vi "_Set Default.vi"   [LabVIEW 2012]
uses:
  <vilib>/eio/EIONode/EIONode.xnode
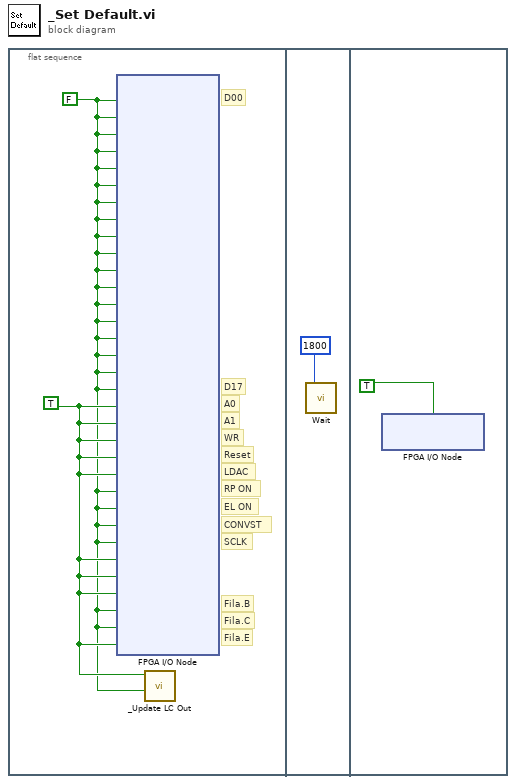
[diagram p0: block diagram]
diagram:
  n1 = flat-sequence {
    frame #0 {
      w2 = TRUE
      w1 = FALSE ("Port4/DIO8")
      # "Fila.E"
      # "Fila.C"
      # "Fila.B"
      # "SCLK"
      # "CONVST"
      # "EL ON"
      # "RP ON"
      # "LDAC"
      # "WR"
      # "A1"
      # "A0"
      # "Reset"
      # "D17"
      # "D00"
      n2 = xnode "FPGA I/O Node"("Port4/DIO8"=w1, "Port4/DIO7"=w1, "Port4/DIO6"=w1, "Port4/DIO5"=w1, "Port4/DIO4"=w1, "Port4/DIO3"=w1, "Port4/DIO2"=w1, "Port4/DIO1"=w1, "Port4/DIO0"=w1, "Port3/DIO8"=w1, "Port3/DIO7"=w1, "Port3/DIO6"=w1, "Port3/DIO5"=w1, "Port3/DIO4"=w1, "Port3/DIO3"=w1, "Port3/DIO2"=w1, "Port3/DIO1"=w1, "Port3/DIO0"=w1, "Port7/DIO1"=w2, "Port7/DIO0"=w2, "Port7/DIO3"=w2, "Port1/DIO4"=w2, "Port7/DIO2"=w2, "Port1/DIO9"=w1, "Port2/DIO9"=w1, "Port6/DIO4"=w1, "Port6/DIO5"=w1, "Port5/DIO1"=w2, "Port5/DIO3"=w2, "Port6/DIO2"=w2, "Port2/DIO5"=w1, "Port2/DIO6"=w1, "Port2/DIO7"=w2) -> ()  [unwired: 33 in, 33 out]
      n3 = call "_Update LC Out.vi"("LC Stop"=w1, "LC Hold"=w2) -> ()  [unwired: 6 out]
    }
    frame #1 {
      n4 = call "Wait"("Count(mSec)"=u16 1800) -> ()  [unwired: 1 out]
    }
    frame #2 {
      n5 = xnode "FPGA I/O Node"("Port6/DIO4"=TRUE ("Port4/DIO8")) -> ()  [unwired: 1 in, 1 out]
    }
  }
